vi "SetValue.vi"(8 "error in":errorcluster, 10 "Value":string, 11 "SequenceFullName in":refnum<class "SequenceFullName.lvclass">) -> (0 "error out":errorcluster, 3 "SequenceFullName out":refnum<class "SequenceFullName.lvclass">)   [LabVIEW 2021, in "ProligentXMLGenerator.lvlib" / "SequenceFullName.lvclass"]
uses:
  SequenceFullName.lvclass
  SequenceFullName.lvclass/SequenceFullName.ctl
  <vilib>/regexp/Match Regular Expression.xnode
  NonEmptyString/NonEmptyString.lvclass
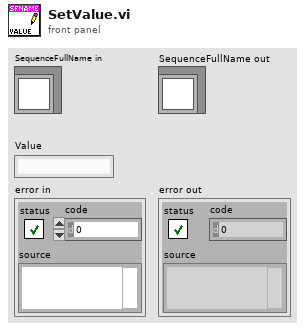
[diagram p1: front panel]
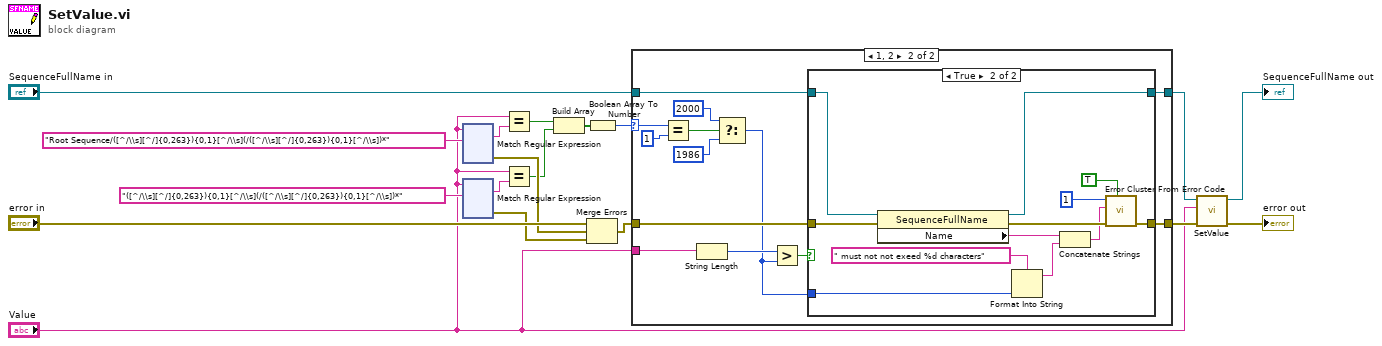
[diagram p0: block diagram]
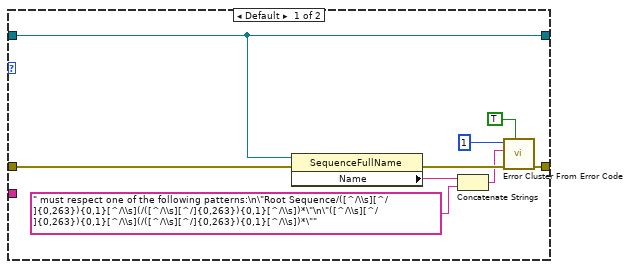
[diagram p2: hidden frame]
diagram:
  n1 = xnode ("Match Regular Expression")("input string"="Value", "regular expression"="Root Sequence/([^/\\s][^/]{0,263}){0,1}[^/\\s](/([^/\\s][^/]{0,263}){0,1}[^/\\s])*") -> ("whole match"=w8:string, "error out"=w5:errorcluster)  [unwired: 4 in, 3 out]
  n2 = xnode ("Match Regular Expression")("input string"="Value", "regular expression"="([^/\\s][^/]{0,263}){0,1}[^/\\s](/([^/\\s][^/]{0,263}){0,1}[^/\\s])*") -> ("whole match"=w12:string, "error out"=w4:errorcluster)  [unwired: 4 in, 3 out]
  n3 = Equal?(x="Value", y=w8) -> (x = y?=w3:bool)
  n4 = Equal?(x="Value", y=w12) -> (x = y?=w2:bool)
  n5 = Build Array(w3, w2) -> (w6:bool[])
  n6 = Merge Errors("error in", w5, w4) -> (w11:errorcluster)
  n7 = Boolean Array To Number(Boolean array=w6) -> (number=w1:u32)
  n8 = case shown="1, 2" w1 {
    selector: w1 -> [_ w33]
    tunnel: "SequenceFullName in" -> [w20 w40]
    tunnel: [w21 w38] -> w14
    tunnel: [w20 w36] -> w13
    tunnel: "Value" -> [_ w35]
    tunnel: w11 -> [w22 w34]
    frame Default {
      n9 = property on="Property Node" class="SequenceFullName"(reference=w20, error in=w22) -> (error out=w26:errorcluster, "Name"=w27:string)  [unwired: 1 out]
      n10 = Concatenate Strings(w27, " must respect one of the following patterns:\n\"Root Sequence/([^/\\s][^/]{0,263}){0,1}[^/\\s](/([^/\\s][^/]{0,263}){0,1}[^/\\s])*\"\n\"([^/\\s][^/]{0,263}){0,1}[^/\\s](/([^/\\s][^/]{0,263}){0,1}[^/\\s])*\"" ("string")) -> (w25:string)
      n11 = call <vilib>:"Error Cluster From Error Code.vi"("show call chain? (False)"=TRUE, "error in (no error)"=w26, "error message (\"\")"=w25, "error code (0)"=1) -> ("error out"=w21:errorcluster)  [unwired: 5 in]
    }
    frame 1, 2 {
      n12 = Equal?(x=w33, y=u32 1) -> (x = y?=w31:bool)
      n13 = String Length(string=w35) -> (length=w39:i32)
      n14 = Select(t=2000 ("y"), s=w31, f=1986 ("y")) -> (s? t:f=w28:i32)
      n15 = Greater?(x=w39, y=w28) -> (0:w37:bool)
      n16 = case shown="True" w37 {
        tunnel: w34 -> [w42 w50]
        tunnel: [w42 w54] -> w38
        tunnel: [w41 w48] -> w36
        tunnel: w40 -> [w41 w51]
        tunnel: w28 -> [_ w43]
        frame False {
        }
        frame True {
          n17 = property on="Property Node" class="SequenceFullName"(reference=w51, error in=w50) -> (reference out=w48:refnum<class "SequenceFullName.lvclass">, error out=w49:errorcluster, "Name"=w52:string)
          n18 = Format Into String(format string=" must not not exeed %d characters" ("string"), w43) -> (resulting string=w45:string)  [unwired: 2 in, 1 out]
          n19 = Concatenate Strings(w52, w45) -> (w47:string)
          n20 = call <vilib>:"Error Cluster From Error Code.vi"("show call chain? (False)"=TRUE, "error in (no error)"=w49, "error message (\"\")"=w47, "error code (0)"=1) -> ("error out"=w54:errorcluster)  [unwired: 5 in]
        }
      }
    }
  }
  n21 = call-parent "SetValue.vi"("error in"=w14, "Value"="Value", "NonEmptyString in"=w13) -> ("error out"=→"error out":errorcluster, "NonEmptyString out"=→"SequenceFullName out":refnum<class "SequenceFullName.lvclass">)  [unwired: 7 in]
